vi "email sender.vi"(7 "Body":string="It works!", 8 "error in (no error)":errorcluster, 9 "Subject":string="Sending TLS Authenticated Email", 10 "Recipient's Name":string="Jane Doe", 11 "Recipient's Email Address Address":string) -> (0 "error out":errorcluster)   [LabVIEW 2012]
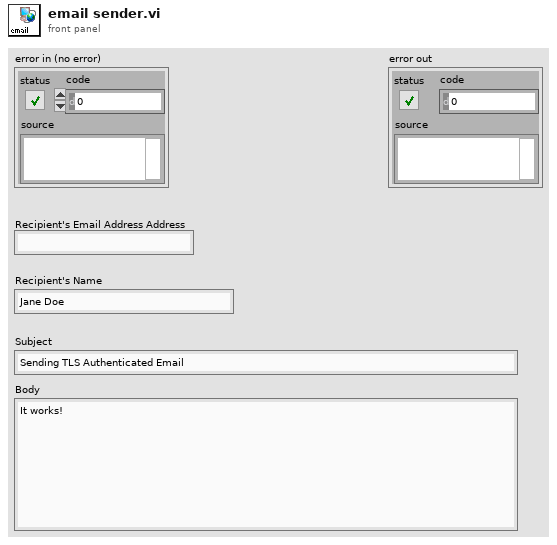
[diagram p1: front panel]
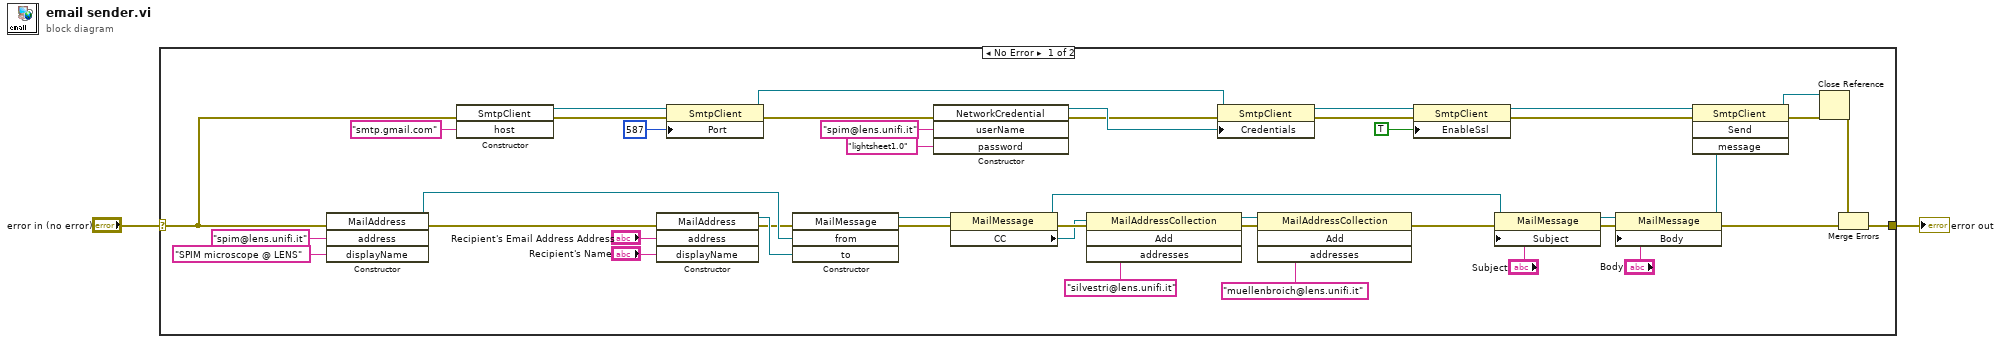
[diagram p0: block diagram]
diagram:
  n1 = case shown="No Error" "error in (no error)" {
    selector: "error in (no error)" -> [w14 w47]
    tunnel: [w3 w47] -> w1
    frame No Error {
      n2 = constructor class="MailAddress"(error in=w14, "address"="spim@lens.unifi.it" ("Sender's Email Address (eg: jsmith77@gmail.com)"), "displayName"="SPIM microscope @ LENS" ("Sender's Name")) -> (reference out=w45:refnum<k24>, error out=w16:errorcluster)  [unwired: 2 in, 3 out]
      n3 = constructor class="SmtpClient"(error in=w14, "host"="smtp.gmail.com" ("Outgoing Mail Server (SMTP)")) -> (reference out=w30:refnum<k24>, error out=w26:errorcluster)  [unwired: 2 in, 2 out]
      n4 = constructor class="MailAddress"(error in=w16, "address"="Recipient's Email Address Address", "displayName"="Recipient's Name") -> (reference out=w46:refnum<k24>, error out=w15:errorcluster)  [unwired: 2 in, 3 out]
      n5 = property class="SmtpClient"(reference=w30, error in=w26, "Port"=587) -> (reference out=w29:refnum<k24>, error out=w13:errorcluster)
      n6 = constructor class="MailMessage"(error in=w15, "from"=w45, "to"=w46) -> (reference out=w21:refnum<k24>, error out=w20:errorcluster)  [unwired: 2 in, 3 out]
      n7 = constructor class="NetworkCredential"(error in=w13, "userName"="spim@lens.unifi.it" ("GMAIL Account User ID (eg: jsmity77)"), "password"="lightsheet1.0" ("GMAIL Account Password")) -> (reference out=w31:refnum<k24>, error out=w12:errorcluster)  [unwired: 2 in, 3 out]
      n8 = property class="MailMessage"(reference=w21, error in=w20) -> (reference out=w19:refnum<k24>, error out=w11:errorcluster, "CC"=w10:refnum<k24>)
      n9 = invoke class="MailAddressCollection" method="Add"(reference=w10, error in=w11, "addresses"="silvestri@lens.unifi.it" ("CC (Carbon Copy Recipient - Optional)")) -> (reference out=w7:refnum<k24>, error out=w9:errorcluster)  [unwired: 1 in, 2 out]
      n10 = property class="SmtpClient"(reference=w29, error in=w12, "Credentials"=w31) -> (reference out=w28:refnum<k24>, error out=w25:errorcluster)
      n11 = invoke class="MailAddressCollection" method="Add"(reference=w7, error in=w9, "addresses"="muellenbroich@lens.unifi.it" ("CC (Carbon Copy Recipient - Optional)")) -> (error out=w8:errorcluster)  [unwired: 1 in, 3 out]
      n12 = property class="SmtpClient"(reference=w28, error in=w25, "EnableSsl"=TRUE ("Enable SSL")) -> (reference out=w27:refnum<k24>, error out=w24:errorcluster)
      n13 = property class="MailMessage"(reference=w19, error in=w8, "Subject"="Subject") -> (reference out=w36:refnum<k24>, error out=w44:errorcluster)
      n14 = property class="MailMessage"(reference=w36, error in=w44, "Body"="Body") -> (reference out=w23:refnum<k24>, error out=w4:errorcluster)
      n15 = invoke class="SmtpClient" method="Send"(reference=w27, error in=w24, "message"=w23) -> (reference out=w18:refnum<k24>, error out=w17:errorcluster)  [unwired: 1 in, 2 out]
      n16 = Close Reference(reference=w18, error in (no error)=w17) -> (error out=w5:errorcluster)
      n17 = Merge Errors(w5, w4) -> (w3:errorcluster)
    }
    frame Error {
    }
  }
  "error out" <- w1
